vi "SelectSpecFile.vi"() -> ()   [LabVIEW 2022 SP3, in "Medulla_ATE.lvlib" / "Medulla_ATE.lvclass"]
uses:
  Medulla_ATE.lvclass
panel:
  out "appended path":path
  out "cancelled":bool
  in  "Path":path
  in  "OK":bool caption="Blank"
  in  "Cancel":bool caption="Blank"
  in  "Select Spec":i32(listbox)
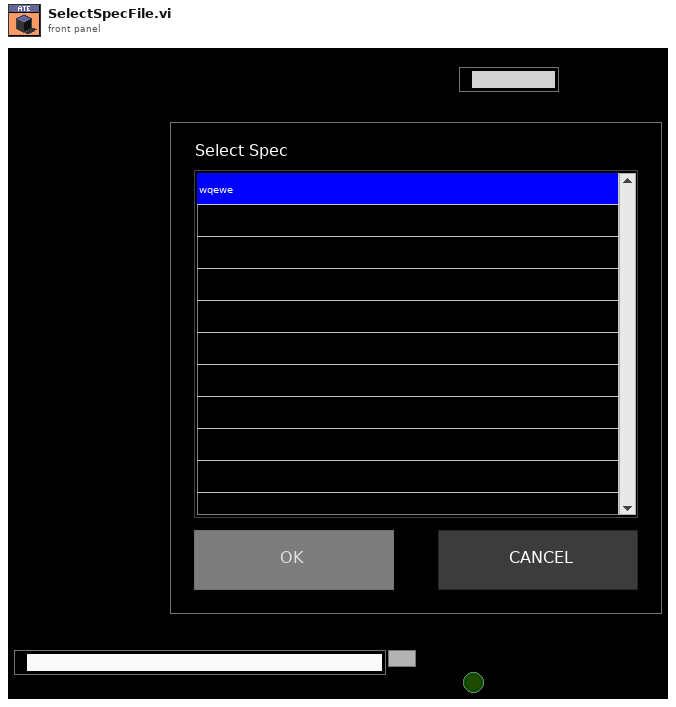
[diagram p1: front panel]
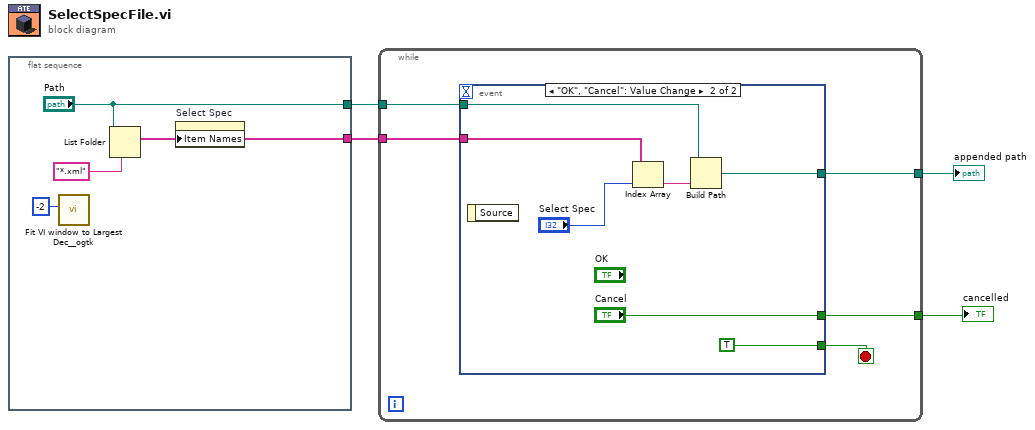
[diagram p0: block diagram]
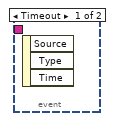
[diagram p2: hidden frame]
diagram:
  n1 = flat-sequence {
    tunnel: [w6] -> w3
    tunnel: ["Path"] -> w2
    frame #0 {
      n2 = call <userlib>:"Fit VI window to Largest Dec__ogtk.vi"("border spacing (2 px)"=-2) -> ()  [unwired: 5 in, 2 out]
      n3 = List Folder(path="Path", pattern="*.xml") -> (filenames=w6:string[])  [unwired: 2 in, 3 out]
      n4 = property on="Select Spec" class="LstBox (strict)"("Item Names"=w6) -> ()  [unwired: 2 in, 2 out]
    }
  }
  n5 = while {
    tunnel: [w13] -> w4
    tunnel: w3 -> [w11]
    tunnel: w2 -> [w10]
    tunnel: [w9] -> w1
    stop <- w12 stop-if-true
    n6 = event shown="[1] \"OK\", \"Cancel\": Value Change" {
      selector: _ -> [_ _]
      dyn-events: _ -> [_ _]
      timeout: _ -> [_ _]
      tunnel: [_ "Cancel"] -> w13
      tunnel: [_ TRUE] -> w12
      tunnel: w11 -> [_ w17]
      tunnel: w10 -> [_ w16]
      tunnel: [_ w14] -> w9
      event Timeout {
        n7 = event-data() -> ()  [unwired: 1 in, 3 out]
      }
      event "OK", "Cancel": Value Change {
        n8 = event-data() -> ()  [unwired: 1 in, 1 out]
        n9 = Index Array(array=w17, index="Select Spec") -> (element=w15:string)
        n10 = Build Path(base path=w16, name or relative path=w15) -> (appended path=w14:path)
      }
    }
  }
  "cancelled" <- w4
  "appended path" <- w1
